vi "singleFreqMultiSwitchMode.vi"(0 "单片机串口":refnum<visa-resource-name>) -> (1 "单片机串口 2":refnum<visa-resource-name>, 2 "I":dbl[](array[numeric]), 3 "Q":dbl[](array[numeric]))   [LabVIEW 2018]
uses:
  PCI8552B_32.dll
panel:
  out "待读取数据长度":i32
  out "当前开关":dbl
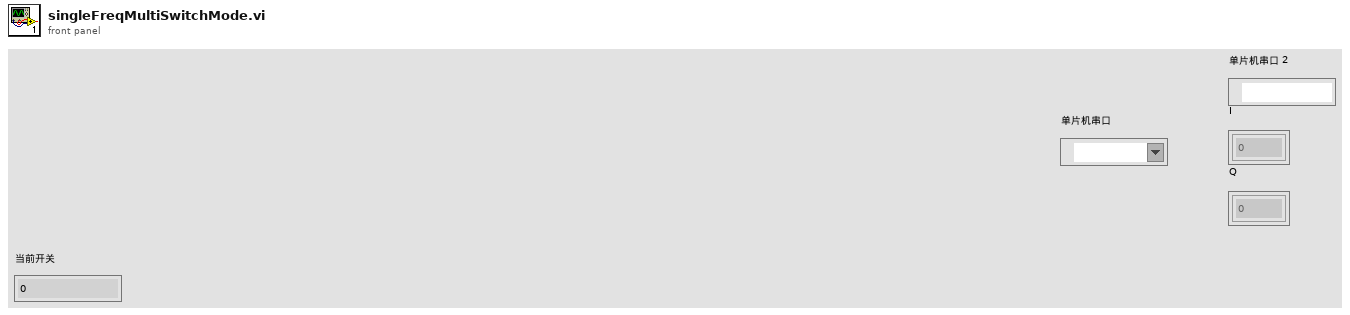
[diagram p1: front panel]
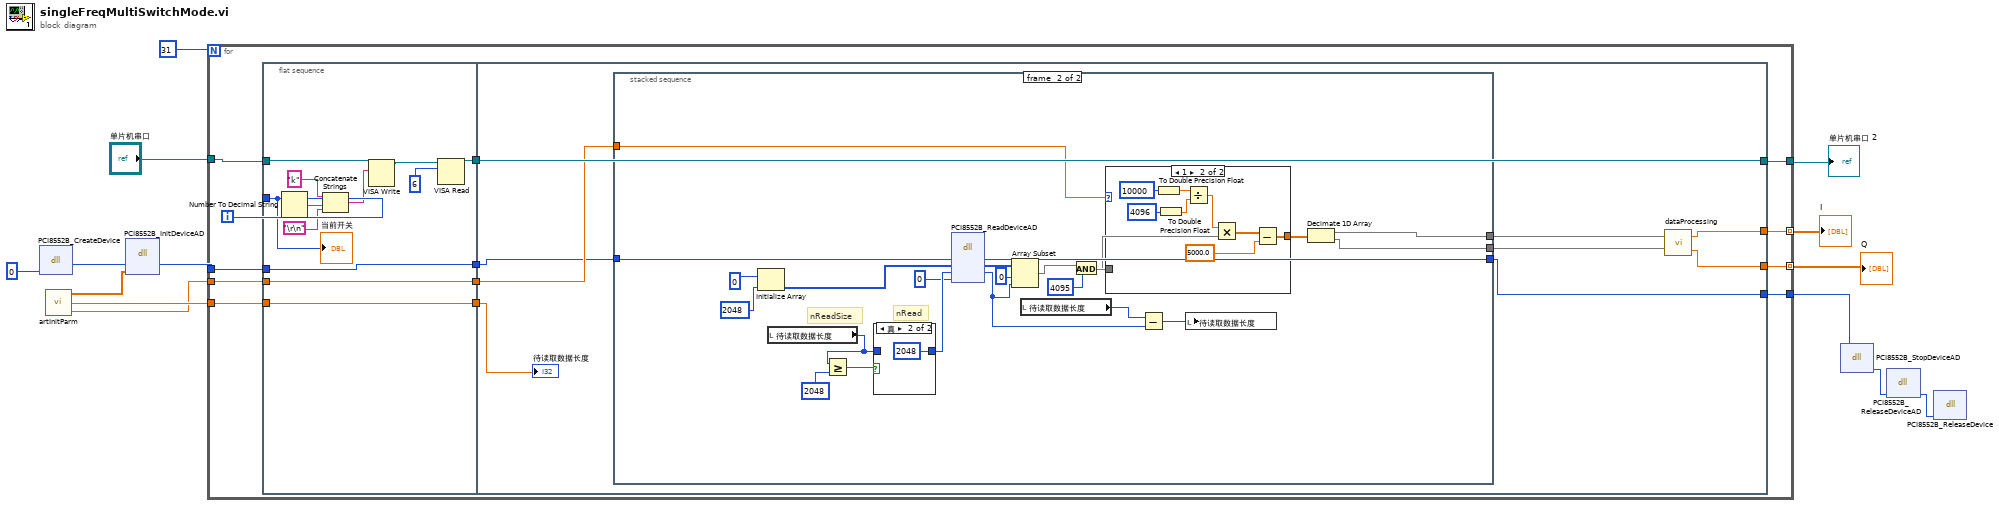
[diagram p0: block diagram]
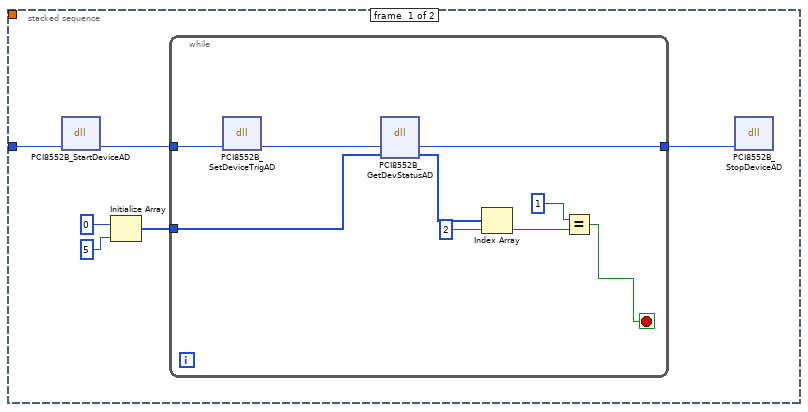
[diagram p2: hidden frame]
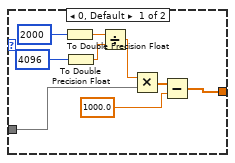
[diagram p3: hidden frame]
diagram:
  n1 = dll-call lib="PTH2€abs E\nPersonal Fileç ”ç©¶ç”Ÿå­¦ä¹ 202002-202007ç ”ä¸€ä¸‹å­¦æœŸwork2020MMW Controllermmw_controllerPCI8552B_32.dll" fn="PCI8552B_CreateDevice" label="CreateDevice"("DeviceLgcID"=0) -> ("返回类型"=w12:i32)  [unwired: 4 in, 2 out]
  n2 = call "artInitParm.vi"() -> ("待读取长度"=w8:dbl, "量程选择"=w9:dbl, "初始化参数"=w13:dbl[])
  n3 = dll-call lib="PTH2€abs E\nPersonal Fileç ”ç©¶ç”Ÿå­¦ä¹ 202002-202007ç ”ä¸€ä¸‹å­¦æœŸwork2020MMW Controllermmw_controllerPCI8552B_32.DLL" fn="PCI8552B_InitDeviceAD" label="InitDeviceAD"("hDevice"=w12, "pADPara"=w13) -> ("hDevice"=w10:i32)  [unwired: 5 in, 2 out]
  n4 = for {
    N: 31 -> [_]
    tunnel: "单片机串口" -> [w27]
    tunnel: [w26] -> w1
    tunnel: w10 -> [w22]
    tunnel: w8 -> [w20]
    tunnel: w9 -> [w18]
    tunnel: [w17] -> w4
    tunnel: [w16] -> w3 mode=indexing
    tunnel: [w15] -> w2 mode=indexing
    i -> [w25]
    n5 = flat-sequence {
      tunnel: w27 -> [w39]
      tunnel: w25 -> [w31]
      tunnel: [w34] -> w24
      tunnel: [w30] -> w23
      tunnel: w22 -> [w30]
      tunnel: [w29] -> w21
      tunnel: w20 -> [w29]
      tunnel: [w28] -> w19
      tunnel: w18 -> [w28]
      tunnel: [w48] -> w26
      tunnel: w24 -> [w48]
      tunnel: w23 -> [w46]
      tunnel: w21 -> [w47]
      tunnel: w19 -> [w45]
      tunnel: [w44] -> w17
      tunnel: [w43] -> w16
      tunnel: [w42] -> w15
      frame #0 {
        n6 = Number To Decimal String(number=w31) -> (decimal integer string=w38:string)  [unwired: 1 in]
        n7 = Concatenate Strings("k", w38, "\r\n") -> (w35:string)
        n8 = VISA Write(VISA resource name=w39, write buffer=w35) -> (VISA resource name out=w33:refnum<visa-resource-name>)  [unwired: 1 in, 2 out]
        n9 = VISA Read(VISA resource name=w33, byte count=6) -> (VISA resource name out=w34:refnum<visa-resource-name>)  [unwired: 1 in, 3 out]
        "当前开关" <- w31
      }
      frame #1 {
        n10 = stacked-sequence {
          tunnel: w46 -> [w50 w81]
          tunnel: [_ w85] -> w44
          tunnel: w47 -> [_ w80]
          tunnel: [_ w79] -> w40
          tunnel: [_ w78] -> w41
          frame #0 {
            n11 = dll-call lib="PTH2€abs E\nPersonal Fileç ”ç©¶ç”Ÿå­¦ä¹ 202002-202007ç ”ä¸€ä¸‹å­¦æœŸwork2020MMW Controllermmw_controllerPCI8552B_32.DLL" fn="PCI8552B_StartDeviceAD" label="StartDeviceAD"("hDevice"=w50) -> ("hDevice"=w49:i32)  [unwired: 4 in, 2 out]
            n12 = Initialize Array(0, 5) -> (w54:i32[])
            n13 = while {
              tunnel: w49 -> [w58]
              tunnel: w54 -> [w63]
              tunnel: [w56] -> w51
              stop <- w55 stop-if-true
              n14 = dll-call lib="PTH2€abs E\nPersonal Fileç ”ç©¶ç”Ÿå­¦ä¹ 202002-202007ç ”ä¸€ä¸‹å­¦æœŸwork2020MMW Controllermmw_controllerPCI8552B_32.DLL" fn="PCI8552B_SetDeviceTrigAD" label="SetDeviceTrigAD"("hDevice"=w58) -> ("hDevice"=w57:i32)  [unwired: 4 in, 2 out]
              n15 = dll-call lib="PTH2€abs E\nPersonal Fileç ”ç©¶ç”Ÿå­¦ä¹ 202002-202007ç ”ä¸€ä¸‹å­¦æœŸwork2020MMW Controllermmw_controllerPCI8552B_32.DLL" fn="PCI8552B_GetDevStatusAD" label="GetDevStatusAD"("hDevice"=w57, "ADStatus"=w63) -> ("hDevice"=w56:i32, "ADStatus"=w59:i32[])  [unwired: 4 in, 2 out]
              n16 = Index Array(array=w59, index=2) -> (element=w61:i32)
              n17 = Equal?(x=1, y=w61) -> (x = y?=w55:bool)
            }
            n18 = dll-call lib="PTH2€abs E\nPersonal Fileç ”ç©¶ç”Ÿå­¦ä¹ 202002-202007ç ”ä¸€ä¸‹å­¦æœŸwork2020MMW Controllermmw_controllerPCI8552B_32.DLL" fn="PCI8552B_StopDeviceAD" label="StopDeviceAD"("hDevice"=w51) -> ()  [unwired: 5 in, 2 out]
          }
          frame #1 {
            # "nReadSize"
            # "nRead"
            n19 = Initialize Array(u16 0 ("y"), 2048 ("y")) -> (w82:u16[])
            n20 = local read "待读取数据长度"() -> (w75:i32)
            n21 = Greater Or Equal?(x=w75, y=2048 ("millisecond multiple")) -> (x >= y?=w76:bool)
            n22 = case shown="真" w76 {
              tunnel: [w104 2048 ("millisecond multiple")] -> w72
              tunnel: w75 -> [w104 _]
              frame False {
              }
              frame True {
              }
            }
            n23 = dll-call lib="PTH2€abs E\nPersonal Fileç ”ç©¶ç”Ÿå­¦ä¹ 202002-202007ç ”ä¸€ä¸‹å­¦æœŸwork2020MMW Controllermmw_controllerPCI8552B_32.DLL" fn="PCI8552B_ReadDeviceAD" label="ReadDeviceAD"("hDevice"=w81, "pADBuffer"=w82, "nReadSizeWords"=w72, "nRetSizeWords"=0) -> ("hDevice"=w85:i32, "pADBuffer"=w67:u16[], "nReadSizeWords"=w64:u32)  [unwired: 5 in, 2 out]
            n24 = Array Subset(array=w67, index=0 ("索引"), length=w64) -> (w66:u16[])
            n25 = local read "待读取数据长度"() -> (w74:i32)
            n26 = And(x=w66, y=u16 4095) -> (x .and. y?=w70:u16[])
            n27 = case shown="1" w80 {
              tunnel: w70 -> [w93 w98]
              tunnel: [w86 w97] -> w69
              frame 0, Default {
                n28 = To Double Precision Float(number=2000 ("x")) -> (double precision float=w89:dbl)
                n29 = To Double Precision Float(number=4096) -> (double precision float=w88:dbl)
                n30 = Divide(x=w89, y=w88) -> (x/y=w94:dbl)
                n31 = Multiply(x=w94, y=w93) -> (x*y=w92:dbl[])
                n32 = Subtract(x=w92, y=1000.0) -> (x-y=w86:dbl[])
              }
              frame 1 {
                n33 = To Double Precision Float(number=10000 ("x")) -> (double precision float=w96:dbl)
                n34 = To Double Precision Float(number=4096) -> (double precision float=w100:dbl)
                n35 = Divide(x=w96, y=w100) -> (x/y=w103:dbl)
                n36 = Multiply(x=w103, y=w98) -> (x*y=w102:dbl[])
                n37 = Subtract(x=w102, y=5000.0) -> (x-y=w97:dbl[])
              }
            }
            n38 = Subtract(x=w74, y=w64) -> (x-y=w73:u32)
            n39 = local write "待读取数据长度"(w73) -> ()
            n40 = Decimate 1D Array(w69) -> (w79:dbl[], w78:dbl[])
          }
        }
        n41 = call "dataProcessing.vi"("中频信号"=w41, "参考信号"=w40) -> ("mean_Q"=w42:dbl, "mean_I"=w43:dbl)
        "待读取数据长度" <- w45
      }
    }
  }
  "I" <- w3
  "Q" <- w2
  "单片机串口 2" <- w1
  n42 = dll-call lib="PTH2€abs E\nPersonal Fileç ”ç©¶ç”Ÿå­¦ä¹ 202002-202007ç ”ä¸€ä¸‹å­¦æœŸwork2020MMW Controllermmw_controllerPCI8552B_32.DLL" fn="PCI8552B_StopDeviceAD" label="StopDeviceAD"("hDevice"=w4) -> ("hDevice"=w6:i32)  [unwired: 4 in, 2 out]
  n43 = dll-call lib="PTH2€abs E\nPersonal Fileç ”ç©¶ç”Ÿå­¦ä¹ 202002-202007ç ”ä¸€ä¸‹å­¦æœŸwork2020MMW Controllermmw_controllerPCI8552B_32.DLL" fn="PCI8552B_ReleaseDeviceAD" label="ReleaseDeviceAD"("hDevice"=w6) -> ("hDevice"=w5:i32)  [unwired: 4 in, 2 out]
  n44 = dll-call lib="PTH2€abs E\nPersonal Fileç ”ç©¶ç”Ÿå­¦ä¹ 202002-202007ç ”ä¸€ä¸‹å­¦æœŸwork2020MMW Controllermmw_controllerPCI8552B_32.DLL" fn="PCI8552B_ReleaseDevice" label="ReleaseDevice"("hDevice"=w5) -> ()  [unwired: 5 in, 2 out]
